vi "Get HighLimit.vi"(8 "Error In":errorcluster, 11 "reference in":refnum<class "OD Entry.lvclass">) -> (0 "Error Out":errorcluster, 2 "HighLimit":string, 3 "reference out":refnum<class "OD Entry.lvclass">)   [LabVIEW 2024, in "Electronic Datasheet.lvlib" / "OD Entry.lvclass"]
uses:
  OD Entry.lvclass
  OD Entry.lvclass/OD Entry.ctl
panel:
  out "Defined?":bool
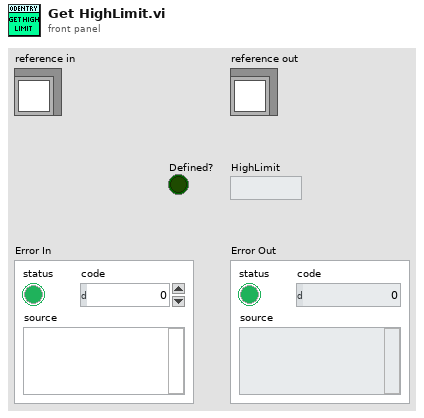
[diagram p1: front panel]
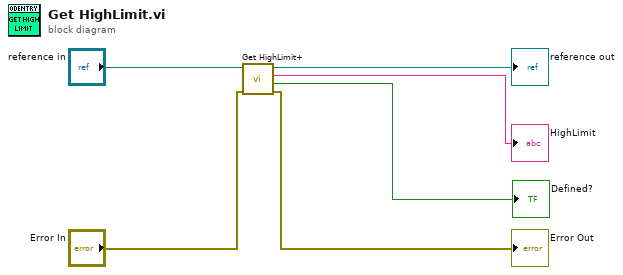
[diagram p0: block diagram]
diagram:
  n1 = call "Get HighLimit+.vi"("Error In"="Error In", "reference in"="reference in") -> ("Error Out"=→"Error Out":errorcluster, "Defined?"=→"Defined?":bool, "HighLimit"=→"HighLimit":string, "reference out"=→"reference out":refnum<class "OD Entry.lvclass">)  [unwired: 6 in]
